vi "FindStringFromEnd.vi"(1 "regular expression":string, 2 "Full String":string) -> (0 "Remaining String":string)   [LabVIEW 2012]
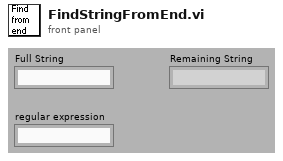
[diagram p1: front panel]
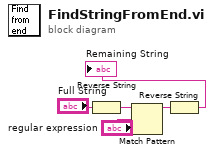
[diagram p0: block diagram]
diagram:
  n1 = Reverse String(1:"Full String") -> (0:w1:string)
  n2 = Match Pattern(string=w1, regular expression="regular expression") -> (before substring=w3:string)  [unwired: 4 out]
  n3 = Reverse String(1:w3) -> (0:→"Remaining String":string)
